vi "6-3.vi"() -> ()   [LabVIEW 2017]
uses:
  <vilib>/Utility/file.llb/Write Delimited Spreadsheet (DBL).vi
  <vilib>/measure/NI_MABase.lvlib
panel:
  out "Y":dbl[](array[numeric])
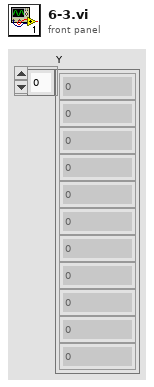
[diagram p1: front panel]
types:
  T1 = enum16{"open", "replace", "create", "open or create", "replace or create", "replace or create with confirmation"}
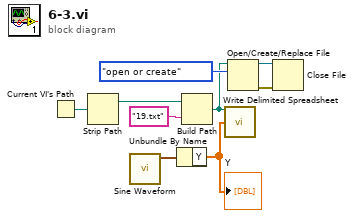
[diagram p0: block diagram]
diagram:
  n1 = Current VI's Path() -> (path=w7:path)
  n2 = Strip Path(path=w7) -> (stripped path=w8:path)  [unwired: 1 out]
  n3 = call <vilib>:"Sine Waveform.vi"() -> ("signal out"=w9:waveform(dbl))  [unwired: 10 in, 1 out]
  n4 = Unbundle By Name(w9) -> ("Y"=w3:dbl[])
  "Y" <- w3
  n5 = Build Path(base path=w8, name or relative path="19.txt" ("名称或相对路径")) -> (appended path=w4:path)
  n6 = call-poly <vilib>:"Write Delimited Spreadsheet.vi"("file path (dialog if empty)"=w4, "1D data"=w3) -> ()  [unwired: 12 in, 2 out]
  n7 = Open/Create/Replace File(file path (use dialog)=w4, operation (0:open)=T1."open or create" ("操作(0:open)")) -> (refnum out=w2:refnum<file>, error out=w1:errorcluster)  [unwired: 4 in, 1 out]
  n8 = Close File(refnum=w2, error in=w1) -> ()  [unwired: 2 out]
